vi "Servo MSMT CDMA2K Set RF WFM Parameters.vi"(8 "error in (no error)":errorcluster, 10 "Step In":refnum<k7>, 11 "Servo MSMT in":refnum<class "Servo MSMT.lvclass">) -> (0 "error out":errorcluster, 2 "Step Out":refnum<k7>, 3 "Servo MSMT out":refnum<class "Servo MSMT.lvclass">)   [LabVIEW 2018, in "Servo MSMT.lvlib" / "Servo MSMT.lvclass"]
uses:
  Servo MSMT.lvclass
  C:/Sequence Automation/Plugins/Measurement Interface.lvlibp/Measurement Interface.lvclass
  Plugins/Measurement Interface.lvlibp/Private Methods/Measurement Parameters/Read Measurement Parameters.vi
  Plugins/String Database.lvlibp/String Database.lvclass
  Plugins/TestStand API Tools (TSAT).lvlibp/Step Actions/TSAT Step Actions.lvlib
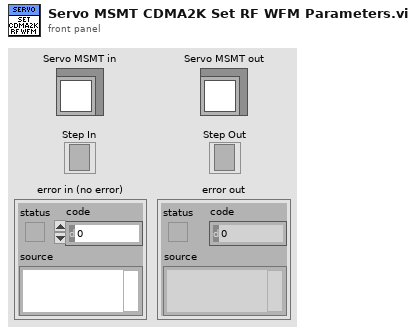
[diagram p1: front panel]
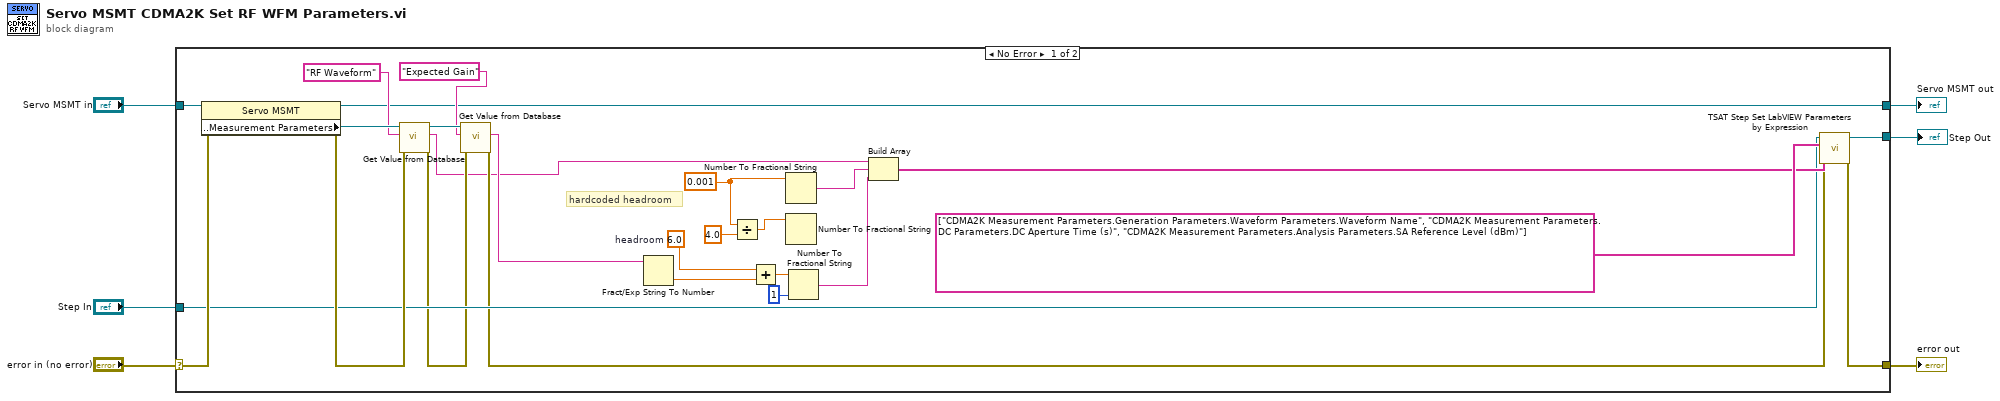
[diagram p0: block diagram]
diagram:
  n1 = case shown="No Error" "error in (no error)" {
    selector: "error in (no error)" -> [w32 w35]
    tunnel: [w29 w35] -> w5
    tunnel: [w10 w34] -> w3
    tunnel: "Servo MSMT in" -> [w28 w34]
    tunnel: [w21 w33] -> w2
    tunnel: "Step In" -> [w20 w33]
    frame No Error {
      w7 = 0.001 ("number")
      w9 = 6.0  # headroom
      # "hardcoded headroom"
      n2 = property class="Servo MSMT"(reference=w28, error in=w32) -> (reference out=w10:refnum<class "Servo MSMT.lvclass">, error out=w26:errorcluster, "Protected Methods:Measurement Parameters"=w27:refnum<class "String Database.lvclass">)
      n3 = call "Get Value from Database.vi"("error in (no error)"=w26, "Entry Name"="RF Waveform", "Message in"=w27) -> ("error out"=w18:errorcluster, "Entry Value"=w8:string, "Message out"=w19:refnum<class "String Database.lvclass">)  [unwired: 5 in, 1 out]
      n4 = call "Get Value from Database.vi"("error in (no error)"=w18, "Entry Name"="Expected Gain", "Message in"=w19) -> ("error out"=w17:errorcluster, "Entry Value"=w15:string)  [unwired: 5 in, 2 out]
      n5 = Fract/Exp String To Number(string=w15) -> (number=w14:dbl)  [unwired: 3 in, 1 out]
      n6 = Divide(x=w7, y=4.0) -> (x/y=w30:dbl)
      n7 = Add(x=w9, y=w14) -> (x+y=w13:dbl)
      n8 = Number To Fractional String(number=w7) -> (F-format string=w24:string)  [unwired: 3 in]
      n9 = Number To Fractional String(number=w30) -> ()  [unwired: 3 in, 1 out]
      n10 = Number To Fractional String(number=w13, precision (6)=i16 1) -> (F-format string=w12:string)  [unwired: 2 in]
      n11 = Build Array(w8, w24, w12) -> (w22:string[])
      n12 = call "TSAT Step Set LabVIEW Parameters by Expression.vi"("Error In"=w17, "Value Expressions"=w22, "Parameters to Set"=string[] ["CDMA2K Measurement Parameters.Generation Parameters.Waveform Parameters.Waveform Name", "CDMA2K Measurement Parameters.DC Parameters.DC Aperture Time (s)", "CDMA2K Measurement Parameters.Analysis Parameters.SA Reference Level (dBm)"], "Step In"=w20) -> ("Error Out"=w29:errorcluster, "Step Out"=w21:refnum<k7>)  [unwired: 6 in]
    }
    frame Error {
    }
  }
  "error out" <- w5
  "Servo MSMT out" <- w3
  "Step Out" <- w2
